vi "VectorNav Read.vi"() -> ()   [LabVIEW 2009]
uses:
  FPGA/VectorNav Heading Global.vi
  <vilib>/rvi/DataTransferAndStorage/Container/XNode/niFpgaContainer.xnode
  <vilib>/rvi/FIFO/Fifo_Resource/nirvififoUniquifyingName.vi
panel:
  out "raw data":u8
  in  "baud rate (9600)":u32=19200
  out "Heading":T1
  out "Number of Elements to Read":u32
types:
  T1 = cluster{"Yaw":fxp<+/-,64,32>, "Pitch":fxp<+/-,64,32>, "Roll":fxp<+/-,64,32>}
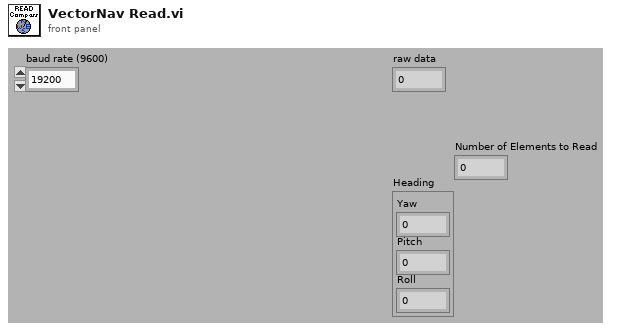
[diagram p1: front panel]
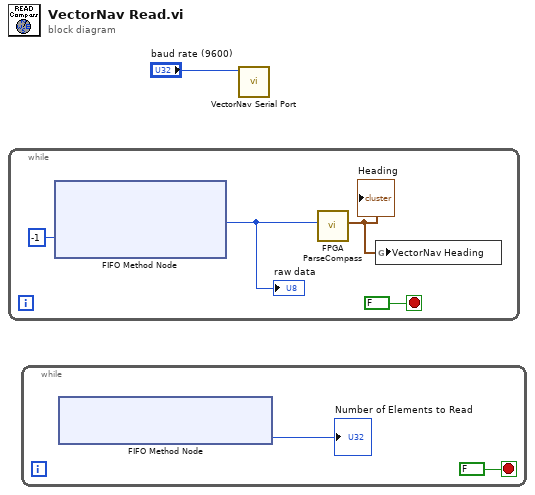
[diagram p0: block diagram]
diagram:
  n1 = while {
    stop <- FALSE stop-if-true
    n2 = xnode ("FIFO Method Node")("Timeout"=-1) -> ("Element"=w5:u8)  [unwired: 1 in, 2 out]
    "raw data" <- w5
    n3 = call "FPGA ParseCompass.vi"("Serial Byte"=w5) -> ("Heading"=w2:T1)  [unwired: 10 in]
    "Heading" <- w2
    n4 = global write "VectorNav Heading Global.vi" "VectorNav Heading"(w2) -> ()
  }
  n5 = while {
    stop <- FALSE stop-if-true
    n6 = xnode ("FIFO Method Node")() -> ("Number of Elements to Read"=→"Number of Elements to Read":u32)  [unwired: 1 in, 1 out]
  }
  n7 = call "VectorNav Serial Port.vi"("baud rate (9600)"="baud rate (9600)") -> ()  [unwired: 11 in]
